vi "Configure Standard Waveform [STD] Core.vi"(4 "dc offset (0.00 V)":dbl[unit] format="%.3f", 5 "start phase (0.00 Degrees)":dbl[unit] format="%.3f", 6 "amplitude (1.00 V)":dbl[unit]=1.0 format="%.3f", 7 "frequency (1000.0 Hz)":dbl[unit]=1000.0 format="%^.2e", 8 "error in (no error)":errorcluster, 9 "waveform (Sine)":i32(ring)=1 items=["Sine"=1, "Square"=2, "Triangle"=3, "Ramp Up"=4, "Ramp Down"=5, "DC"=6], 10 "channel name (\"CHANNEL1\")":string="CHANNEL1", 11 "IVI_Fgen in":refnum<class "IVI_Fgen.lvclass">) -> (0 "error out":errorcluster, 3 "IVI_Fgen out":refnum<class "IVI_Fgen.lvclass">)   [LabVIEW 2013, in "IVI_Fgen.lvlib" / "IVI_Fgen.lvclass"]
doc: "This VI configures the properties of the function generator that affect standard waveform generation. These properties are the waveform, amplitude, DC offset, frequency, and start phase.\n\nNotes:\n\n(1) This VI is part of the IviFgenStdFunc [STD] extension group."
uses:
  IVI_Fgen.lvclass
  IVI_Fgen.lvclass/IVI_Fgen.ctl
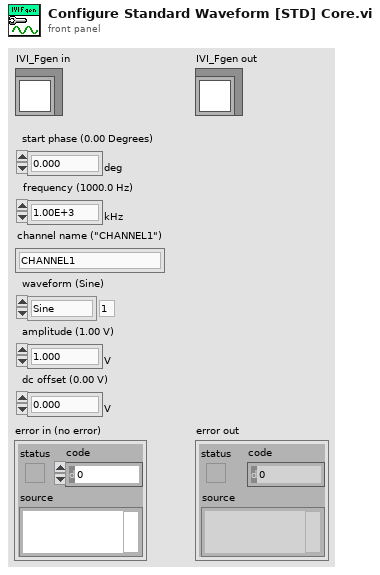
[diagram p1: front panel]
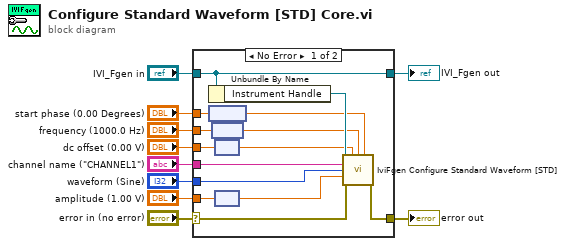
[diagram p0: block diagram]
diagram:
  n1 = case shown="No Error" "error in (no error)" {
    selector: "error in (no error)" -> [w22 w26]
    tunnel: [w21 w26] -> w9
    tunnel: [w24 w25] -> w7
    tunnel: "IVI_Fgen in" -> [w24 w25]
    tunnel: "channel name (\"CHANNEL1\")" -> [w20 _]
    tunnel: "start phase (0.00 Degrees)" -> [w19 _]
    tunnel: "frequency (1000.0 Hz)" -> [w18 _]
    tunnel: "dc offset (0.00 V)" -> [w17 _]
    tunnel: "waveform (Sine)" -> [w16 _]
    tunnel: "amplitude (1.00 V)" -> [w15 _]
    frame No Error {
      n2 = Unbundle By Name(w24) -> ("Instrument Handle"=w23:refnum<k15>)
      n3 = node(w19) -> (w14:dbl)
      n4 = node(w18) -> (w13:dbl)
      n5 = node(w17) -> (w12:dbl)
      n6 = node(w15) -> (w11:dbl)
      n7 = call <vilib>:"IviFgen Configure Standard Waveform [STD].vi"("instrument handle"=w23, "dc offset (0.00 V)"=w12, "frequency (1000.0 Hz)"=w13, "start phase (0.00 Degrees)"=w14, "channel name (\"CHANNEL1\")"=w20, "waveform (Sine)"=w16, "amplitude (1.00 V)"=w11, "error in (no error)"=w22) -> ("error out"=w21:errorcluster)  [unwired: 6 in, 1 out]
    }
    frame Error {
    }
  }
  "error out" <- w9
  "IVI_Fgen out" <- w7
